vi "Teleop.vi"(10 "Match Info":T4={"Autonomous Elapsed Seconds"=0.0, "TeleOp Elapsed Seconds"=0.0, "Disabled Elapsed Seconds"=0.0, "Visited Autonomous"=FALSE, "Visited TeleOp"=FALSE, "Visited Disabled"=FALSE, "Autonomous Settings"={"Autonomous Style"=enum."Independent", "VI Refnum"=refnum}}, 11 "Call Context":T5) -> ()   [LabVIEW 2018]
doc: "This VI is called for each TeleOp packet received from the DS where the robot is not disabled. It is often used to read from the joysticks and update I/O or to update setpoints for timed control loops. It should complete and return within 20 milliseconds or it may miss DS packets."
uses:
  <vilib>/Rock Robotics/WPI/DriverStation/WPI_DriverStationDerivedRobotMode.ctl
  <vilib>/Rock Robotics/WPI/DriverStation/WPI_DriverStationMatch Info.ctl
  Typedefs/typedef_cluster_TeleOp_Local_Data.ctl
  Typedefs/typedef_cluster_Joystick.ctl
  Typedefs/typedef_cluster_Vision.ctl
  Typedefs/typedef_enum_TeleOp_State.ctl
panel:
  out "error out":errorcluster
  out "Teleop Local Data":T1 {"Vision"."Theta_Y" format="%.1f"; "Vision"."Theta_X" format="%.1f"; "Potentio" format="%.1f"; "Drive_Enc_R" format="%.1f"; "Drive_Enc_L" format="%.1f"; "Gyro_Angle" format="%.1f"; "Encoder_Lift" format="%.1f"; "Motor_Lift" format="%.3f"; "Motor_Intake" format="%.3f"; "Drive_Twist" format="%.3f"; "Drive_Forward" format="%.3f"}
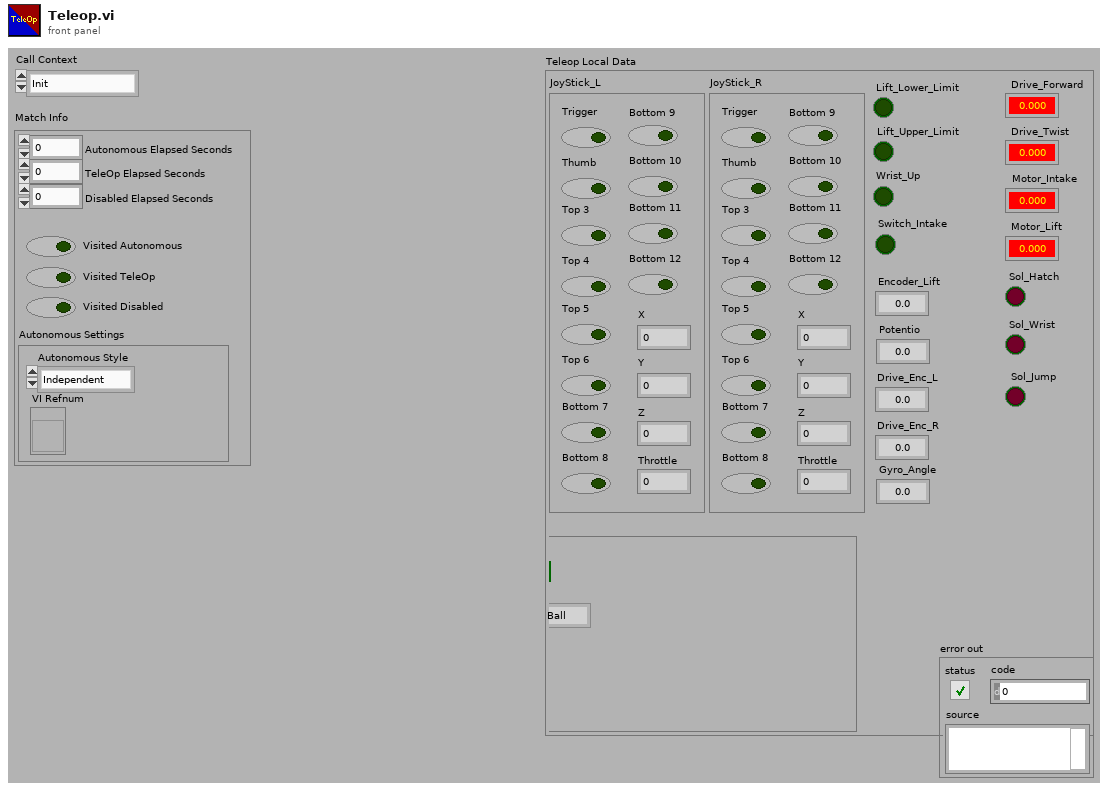
[diagram p1: front panel]
types:
  T1 = typedef "typedef_cluster_TeleOp_Local_Data.ctl" = cluster{"Lift_Lower_Limit":bool, "Wrist_Up":bool, "Switch_Intake":bool, "Encoder_Lift":dbl, "Sol_Wrist":bool, "Motor_Intake":dbl, "Motor_Lift":dbl, "Drive_Forward":dbl, "Drive_Twist":dbl, "Sol_Hatch":bool, "Gyro_Angle":dbl, "Drive_Enc_L":dbl, "Drive_Enc_R":dbl, "JoyStick_L":T2, "JoyStick_R":T2, "Potentio":dbl, "Vision":T3, "Lift_Upper_Limit":bool, "Sol_Jump":bool}
  T2 = typedef "typedef_cluster_Joystick.ctl" = cluster{"X":dbl, "Y":dbl, "Z":dbl, "Throttle":dbl, "Trigger":bool, "Thumb":bool, "Top 3":bool, "Top 4":bool, "Top 5":bool, "Top 6":bool, "Bottom 7":bool, "Bottom 8":bool, "Bottom 9":bool, "Bottom 10":bool, "Bottom 11":bool, "Bottom 12":bool}
  T3 = typedef "typedef_cluster_Vision.ctl" = cluster{"Theta_X":dbl, "Theta_Y":dbl, "Has_Target":bool, "Seek_Ball":bool, "Pipeline":enum16{"Ball", "Dual_Target", "Single_Target"}}
  T4 = typedef "WPI_DriverStationMatch Info.ctl" = cluster{"Autonomous Elapsed Seconds":dbl, "TeleOp Elapsed Seconds":dbl, "Disabled Elapsed Seconds":dbl, "Visited Autonomous":bool, "Visited TeleOp":bool, "Visited Disabled":bool, "Autonomous Settings":cluster{"Autonomous Style":enum16{"Iterative", "Independent"}, "VI Refnum":refnum<vi>}}
  T5 = typedef "WPI_DriverStationDerivedRobotMode.ctl" = enum16{"Init", "Execute", "Stop"}
  T6 = typedef "typedef_enum_TeleOp_State.ctl" = enum16{"Read NT", "Read Joy", "Read Gyro", "Read Drive Encoders", "Read Limit", "Calc Vision", "Calc Wrist", "Calc Drive", "Calc Fly", "Calc Lift", "Calc Hatch", "Write Wrist", "Write Drive", "Write Fly", "Write Lift", "Write Hatch", "Write Jump", "Write NT"}
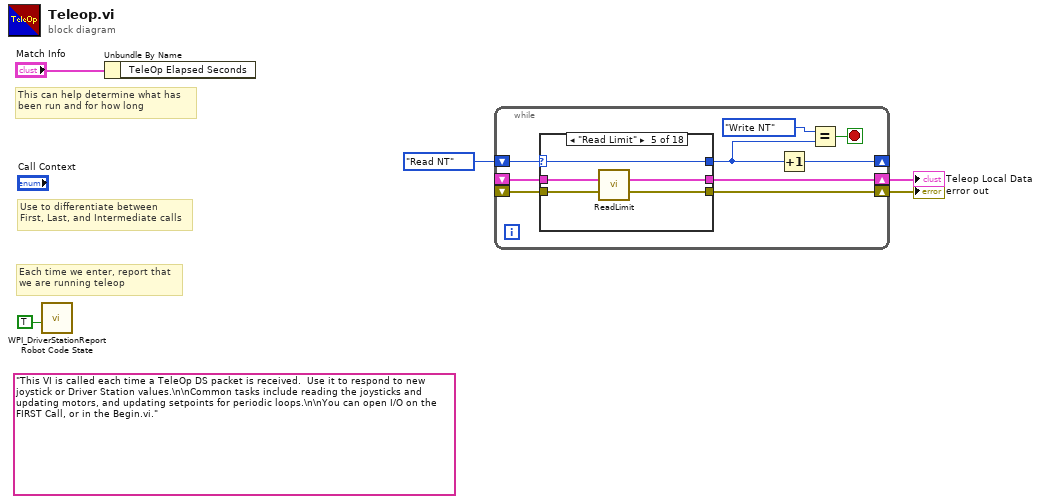
[diagram p0: block diagram]
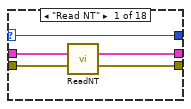
[diagram p2: hidden frame]
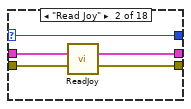
[diagram p3: hidden frame]
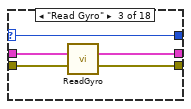
[diagram p4: hidden frame]
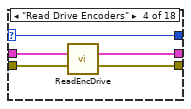
[diagram p5: hidden frame]
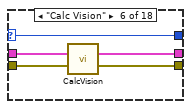
[diagram p6: hidden frame]
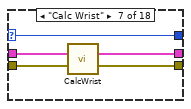
[diagram p7: hidden frame]
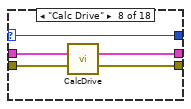
[diagram p8: hidden frame]
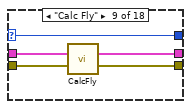
[diagram p9: hidden frame]
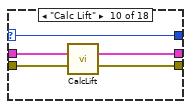
[diagram p10: hidden frame]
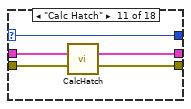
[diagram p11: hidden frame]
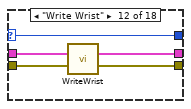
[diagram p12: hidden frame]
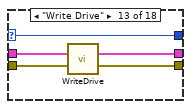
[diagram p13: hidden frame]
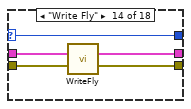
[diagram p14: hidden frame]
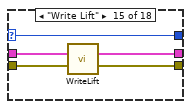
[diagram p15: hidden frame]
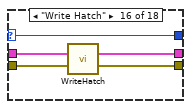
[diagram p16: hidden frame]
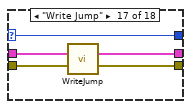
[diagram p17: hidden frame]
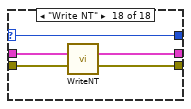
[diagram p18: hidden frame]
diagram:
  (unwired) "This VI is called each time a TeleOp DS packet is received.  Use it to respond to new joystick or Driver Station values.\n\nCommon tasks include reading the joysticks and updating motors, and updating setpoints for periodic loops.\n\nYou can open I/O on the FIRST Call, or in the Begin.vi."
  # "Each time we enter, report that\nwe are running teleop"
  # "Use to differentiate between\nFirst, Last, and Intermediate calls"
  # "This can help determine what has\nbeen run and for how long"
  n1 = call <vilib>:"WPI_DriverStationReport Robot Code State.vi"("TeleOp"=TRUE ("Autonomous")) -> ()  [unwired: 10 in, 1 out]
  n2 = Unbundle By Name("Match Info") -> ()  [unwired: 1 out]
  n3 = while {
    shift-right: [w11] -> _
    shift-left: typedef_enum_TeleOp_State."Read NT" -> [w8]
    shift-right: [w13] -> w2
    shift-left: _ -> [w12]
    shift-right: [w10] -> w1
    shift-left: _ -> [w9]
    stop <- w14 stop-if-true
    n4 = case shown="\"Read Limit\"" w8 {
      selector: w8 -> [w19 w24 w29 w34 w39 w44 w49 w53 w57 w62 w67 w72 w77 w82 w87 w92 w97 w102]
      tunnel: [w19 w24 w29 w34 w39 w44 w49 w53 w57 w62 w67 w72 w77 w82 w87 w92 w97 w102] -> w6
      tunnel: [w15 w21 w27 w32 w35 w41 w46 w50 w55 w59 w64 w69 w74 w79 w84 w89 w95 w98] -> w13
      tunnel: w12 -> [w18 w23 w28 w33 w38 w43 w48 w51 w54 w61 w66 w71 w76 w81 w86 w91 w96 w101]
      tunnel: [w16 w20 w25 w30 w36 w40 w45 w52 w56 w58 w63 w68 w73 w78 w83 w88 w94 w99] -> w10
      tunnel: w9 -> [w17 w22 w26 w31 w37 w42 w47 w52 w56 w60 w65 w70 w75 w80 w85 w90 w93 w100]
      frame "Read NT" {
        n5 = call "ReadNT.vi"("Teleop Local Data"=w18, "error in"=w17) -> ("Teleop Local Data Out"=w15:T1, "error out"=w16:errorcluster)  [unwired: 12 in]
      }
      frame "Read Joy" {
        n6 = call "ReadJoy.vi"("Teleop Local Data Out in"=w23, "error in (no error)"=w22) -> ("Teleop Local Data Out out"=w21:T1, "error out"=w20:errorcluster)  [unwired: 12 in]
      }
      frame "Read Gyro" {
        n7 = call "ReadGyro.vi"("Teleop Local Data"=w28, "error in"=w26) -> ("Out Teleop Local Data"=w27:T1, "error out"=w25:errorcluster)  [unwired: 12 in]
      }
      frame "Read Drive Encoders" {
        n8 = call "ReadEncDrive.vi"("Teleop Local Data"=w33, "error in"=w31) -> ("Teleop Local Data Out"=w32:T1, "error out"=w30:errorcluster)  [unwired: 12 in]
      }
      frame "Read Limit" {
        n9 = call "ReadLimit.vi"("Teleop Local Data In"=w38, "error in"=w37) -> ("Teleop Local Data Out"=w35:T1, "error out"=w36:errorcluster)  [unwired: 12 in]
      }
      frame "Calc Vision" {
        n10 = call "CalcVision.vi"("Teleop Local Data In"=w43, "error in (no error)"=w42) -> ("Teleop Local Data Out"=w41:T1, "error out"=w40:errorcluster)  [unwired: 12 in]
      }
      frame "Calc Wrist" {
        n11 = call "CalcWrist.vi"("Teleop Local Data Out in"=w48, "error in (no error)"=w47) -> ("Teleop Local Data Out out"=w46:T1, "error out"=w45:errorcluster)  [unwired: 12 in]
      }
      frame "Calc Drive" {
        n12 = call "CalcDrive.vi"("Teleop Local Data In"=w51) -> ("Teleop Local Data Out"=w50:T1)  [unwired: 14 in]
      }
      frame "Calc Fly" {
        n13 = call "CalcFly.vi"("Teleop Local Data Out in"=w54) -> ("Teleop Local Data Out out"=w55:T1)  [unwired: 14 in]
      }
      frame "Calc Lift" {
        n14 = call "CalcLift.vi"("Teleop Local Data In"=w61, "error in"=w60) -> ("Teleop Local Data Out"=w59:T1, "error out"=w58:errorcluster)  [unwired: 12 in]
      }
      frame "Calc Hatch" {
        n15 = call "CalcHatch.vi"("Teleop Local Data Out in"=w66, "error in (no error)"=w65) -> ("Teleop Local Data Out out"=w64:T1, "error out"=w63:errorcluster)  [unwired: 12 in]
      }
      frame "Write Wrist" {
        n16 = call "WriteWrist.vi"("Teleop Local Data in"=w71, "error in (no error)"=w70) -> ("Teleop Local Data Out"=w69:T1, "error out"=w68:errorcluster)  [unwired: 12 in]
      }
      frame "Write Drive" {
        n17 = call "WriteDrive.vi"("Teleop Local Data In"=w76, "error in (no error)"=w75) -> ("Teleop Local Data Out"=w74:T1, "error out"=w73:errorcluster)  [unwired: 12 in]
      }
      frame "Write Fly" {
        n18 = call "WriteFly.vi"("Teleop Local Data Out"=w81, "error in (no error)"=w80) -> ("Teleop Local Data Out 2"=w79:T1, "error out"=w78:errorcluster)  [unwired: 12 in]
      }
      frame "Write Lift" {
        n19 = call "WriteLift.vi"("Teleop Local Data"=w86, "error in"=w85) -> ("Teleop Local Data Out"=w84:T1, "error out"=w83:errorcluster)  [unwired: 12 in]
      }
      frame "Write Hatch" {
        n20 = call "WriteHatch.vi"("Teleop Local Data Out"=w91, "error in (no error)"=w90) -> ("Teleop Local Data Out"=w89:T1, "error out"=w88:errorcluster)  [unwired: 12 in]
      }
      frame "Write Jump" {
        n21 = call "WriteJump.vi"("Teleop Local Data In"=w96, "error in"=w93) -> ("Teleop Local Data Out"=w95:T1, "error out"=w94:errorcluster)  [unwired: 12 in]
      }
      frame "Write NT" {
        n22 = call "WriteNT.vi"("Teleop Local Data In"=w101, "error in"=w100) -> ("Teleop Local Data Out"=w98:T1, "error out"=w99:errorcluster)  [unwired: 12 in]
      }
    }
    n23 = Increment(x=w6) -> (x+1=w11:T6)
    n24 = Equal?(x=typedef_enum_TeleOp_State."Write NT" ("y"), y=w6) -> (x = y?=w14:bool)
  }
  "Teleop Local Data" <- w2
  "error out" <- w1
